vi "Ask_NewName.vi"(10 "New Name":string, 11 "Label":string) -> (1 "OK":bool, 3 "New Name out":string caption="New Name")   [LabVIEW 2022 SP3]
panel:
  out "error out":errorcluster
  in  "error in (no error)":errorcluster
  in  "Cancel":bool
  in  "OK ?":bool caption="OK2"
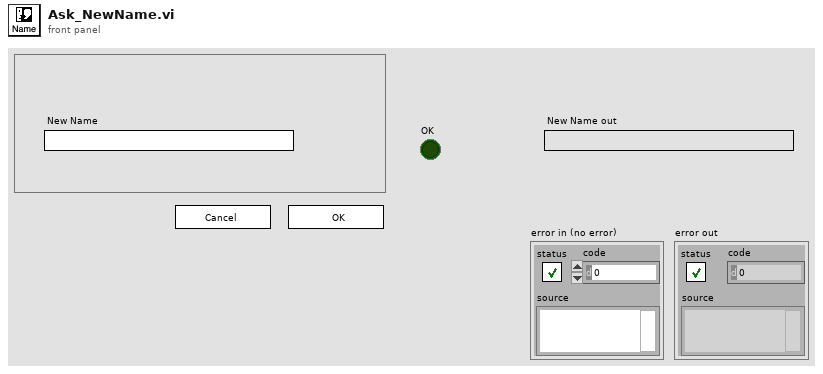
[diagram p1: front panel]
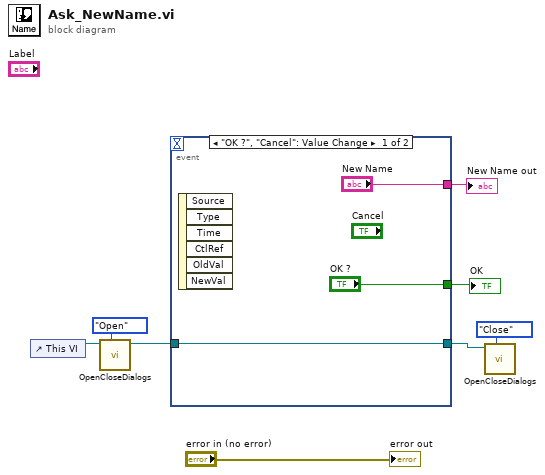
[diagram p0: block diagram]
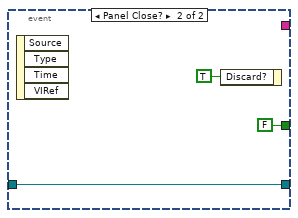
[diagram p2: hidden frame]
diagram:
  n1 = control-ref of="This VI"() -> (w4:refnum<vi>)
  n2 = call "OpenCloseDialogs.vi"("Task"=enum16{"Open", "Close"}."Open", "VI in"=w4) -> ("VI out"=w1:refnum<vi>)  [unwired: 8 in, 1 out]
  n3 = event shown="[0] \"OK ?\", \"Cancel\": Value Change" {
    selector: _ -> [_ _]
    dyn-events: _ -> [_ _]
    timeout: _ -> [_ _]
    tunnel: ["OK ?" FALSE ("OK ?")] -> w8
    tunnel: ["New Name" _] -> w6
    tunnel: [w9 w12] -> w2
    tunnel: w1 -> [w9 w12]
    event "OK ?", "Cancel": Value Change {
      n4 = event-data() -> ()  [unwired: 1 in, 6 out]
    }
    event Panel Close? {
      n5 = event-data() -> ()  [unwired: 1 in, 4 out]
      n6 = event-data("Discard?"=TRUE) -> ()  [unwired: 1 in, 1 out]
    }
  }
  "OK" <- w8
  "New Name out" <- w6
  n7 = call "OpenCloseDialogs.vi"("Task"=enum16{"Open", "Close"}."Close", "VI in"=w2) -> ()  [unwired: 8 in, 2 out]
  "error out" <- "error in (no error)"
